vi "OpenALPR_test_Path.vi"(8 "error in (no error)":errorcluster) -> (0 "error out":errorcluster, 3 "path":string)   [LabVIEW 2014, in "OpenALPR in LabView.lvlib"]
doc: "Send back the path of the openalpr library for test purpose.\n\n\n\n\n\nextern \"C\" __declspec(dllexport) char* test_Path(void);"
uses:
  OpenALPR in LabView.lvlib
  Dlls/OALPRLabVIEW.dll
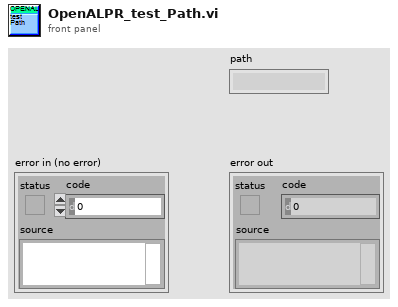
[diagram p1: front panel]
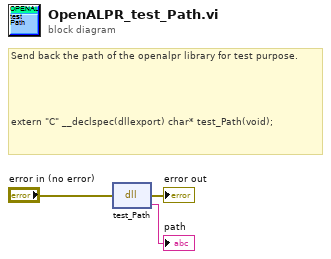
[diagram p0: block diagram]
diagram:
  # "Send back the path of the openalpr library for test purpose.\n\n\n\n\n\nextern \"C\" __declspec(dllexport) char* test_Path(void);"
  n1 = dll-call lib="PTH2abs EFelhasznÃ¡lÃ³kPixelbetyÃ¡rDesktopC19 -C3 Verseny bekÃ¼ldÃ©shez\tSmartMarkOpenALPR to LVOpenALPR_LabVIEWDllsOALPRLabVIEW.*" fn="test_Path"(error in="error in (no error)") -> (error out=→"error out":errorcluster, "return type"=→"path":string)  [unwired: 2 in, 1 out]
